vi "电流测试.vi"(0 "IT6512C":refnum<visa-resource-name>="GPIB0::16::INSTR", 1 "2700":refnum<visa-resource-name>="GPIB0::16::INSTR", 2 "delta":dbl, 3 "start":dbl caption="首端", 4 "end":dbl=1.0 caption="末端", 5 "error in (no error)":errorcluster) -> (13 "error out":errorcluster, 15 "回读电流":dbl[](array[numeric]), 16 "输入电流":dbl[](array[numeric]), 17 "误差":dbl[](array[numeric]), 18 "斜率":dbl, 19 "截距":dbl)   [LabVIEW 2020]
uses:
  <vilib>/Analysis/1siggen.llb/Ramp Pattern by Delta.vi
  <vilib>/Analysis/NI_AALBase.lvlib
  <vilib>/ptbypt/NI_PtbyPt.lvlib
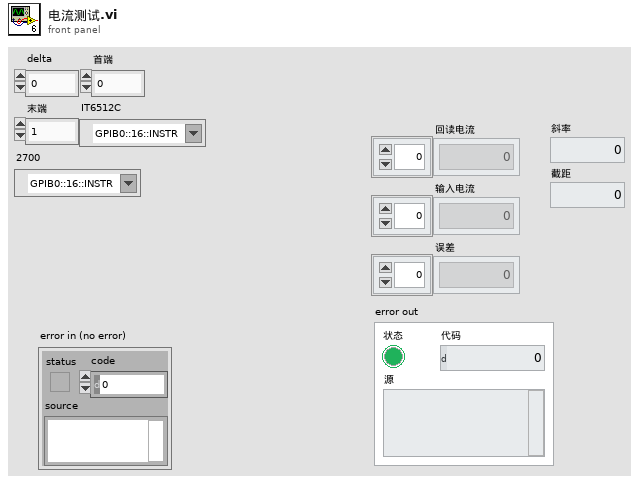
[diagram p1: front panel]
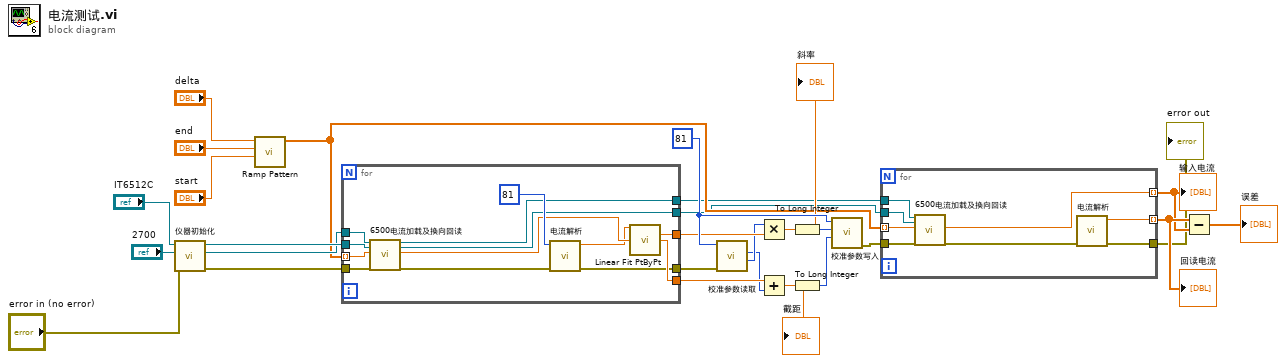
[diagram p0: block diagram]
diagram:
  w19 = u16 81 ("Channel")
  n1 = call "仪器初始化.vi"("error in (no error)"="error in (no error)", "2700"="2700", "IT6512C"="IT6512C") -> ("error out"=w20:errorcluster, "2700"=w23:refnum<visa-resource-name>, "IT6512C"=w24:refnum<visa-resource-name>)  [unwired: 6 in]
  n2 = call-poly <vilib>:"Ramp Pattern.vi"("start"="start", "end"="end", "delta"="delta") -> ("Ramp Pattern"=w12:dbl[])  [unwired: 6 in, 2 out]
  n3 = for {
    tunnel: w12 -> [w38] mode=indexing
    tunnel: w24 -> [w40]
    tunnel: w23 -> [w39]
    tunnel: w20 -> [w36]
    tunnel: [w32] -> w18
    tunnel: [w31] -> w15
    tunnel: [w30] -> w11
    tunnel: [w29] -> w7
    tunnel: [w28] -> w6
    n4 = call "6500电流加载及换向回读.vi"("2700 in"=w39, "IT6512C in"=w40, "输入电流"=w38, "error in"=w36) -> ("2700 out"=w29:refnum<visa-resource-name>, "IT6512C out"=w28:refnum<visa-resource-name>, "实际电流"=w34:dbl, "error out"=w35:errorcluster)  [unwired: 12 in]
    n5 = call "电流解析.vi"("error in"=w35, "Channel"=u16 81) -> ("error out"=w30:errorcluster, "读取电流"=w33:dbl)  [unwired: 8 in]
    n6 = call <vilib>:"Linear Fit PtByPt.vi"("y"=w33, "x"=w34) -> ("slope"=w32:dbl, "intercept"=w31:dbl)  [unwired: 9 in, 3 out]
  }
  n7 = call "校准参数读取.vi"("error in"=w11, "Channel"=w19) -> ("斜率"=w10:i32, "截距"=w9:i32)  [unwired: 7 in, 1 out]
  n8 = Multiply(x=w10, y=w18) -> (x*y=w17:dbl)
  "斜率" <- w17
  n9 = Add(x=w15, y=w9) -> (x+y=w14:dbl)
  "截距" <- w14
  n10 = To Long Integer(number=w17) -> (32bit integer=w16:i32)
  n11 = To Long Integer(number=w14) -> (32bit integer=w13:i32)
  n12 = call "校准参数写入.vi"("截距"=w13, "斜率"=w16, "Channel"=w19) -> ("error out"=w8:errorcluster)  [unwired: 7 in, 1 out]
  n13 = for {
    tunnel: w12 -> [w44] mode=indexing
    tunnel: w8 -> [w47]
    tunnel: w7 -> [w46]
    tunnel: w6 -> [w45]
    tunnel: [w43] -> w5 mode=indexing
    tunnel: [w42] -> w4 mode=indexing
    tunnel: [w41] -> w1
    n14 = call "6500电流加载及换向回读.vi"("2700 in"=w46, "IT6512C in"=w45, "输入电流"=w44, "error in"=w47) -> ("实际电流"=w42:dbl, "error out"=w48:errorcluster)  [unwired: 12 in, 2 out]
    n15 = call "电流解析.vi"("error in"=w48) -> ("error out"=w41:errorcluster, "读取电流"=w43:dbl)  [unwired: 9 in]
  }
  "回读电流" <- w5
  "输入电流" <- w4
  "error out" <- w1
  n16 = Subtract(x=w5, y=w4) -> (x-y=→"误差":dbl[])
